vi "make_stim_protocol.vi"(8 "Error in":errorcluster, 10 "Device parameters":T1={"Triggered?"=FALSE, "Shutter channel"="", "Acquisition channels"="", "Acquisition sample rate"=1000.0, "Read chunk size"=100, "Stimulation channel"="Dev1/ao0", "Stimulation sample rate"=100.0} {"Read chunk size" min=100 max=100000; "Acquisition sample rate" min=10.0 max=10000.0 step=10.0; "Stimulation sample rate" min=10.0 max=10000.0}, 11 "Protocol parameters":T2={"Repetitions"=1.0, "ON time"=40.0, "OFF time"=120.0, "Stim onset"=5.0, "Stim frequency"=1.0, "Pulse width"=1.0, "Acquire before ON"=1.0, "Acquire after ON"=1.0, "Sync shutter to acquisition"=TRUE} {"Pulse width" min=0.0001 max=0.1 step=0.01; "Acquire after ON" min=0.0 max=10.0 step=1.0; "Acquire before ON" min=0.0 max=10.0 step=1.0; "Repetitions" min=1.0 max=10.0 step=1.0; "OFF time" min=0.0 max=1000.0; "ON time" min=0.0 max=1000.0; "Stim onset" min=0.0 max=6000.0; "Stim frequency" min=-2.0 max=40.0 step=1.0}) -> (0 "Error out":errorcluster, 2 "Stim array":dbl[](array[numeric]))   [LabVIEW 2010]
uses:
  typedefs/protocol_parameters.ctl
  typedefs/device_parameters.ctl
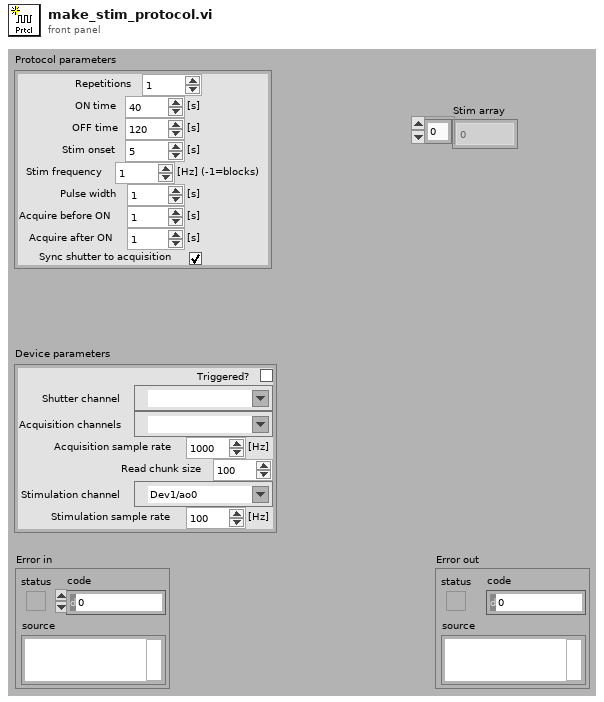
[diagram p1: front panel]
types:
  T1 = typedef "device_parameters.ctl" = cluster{"Triggered?":bool, "Shutter channel":tag, "Acquisition channels":tag, "Acquisition sample rate":dbl, "Read chunk size":i32, "Stimulation channel":tag, "Stimulation sample rate":dbl}
  T2 = typedef "protocol_parameters.ctl" = cluster{"Repetitions":dbl, "ON time":dbl, "OFF time":dbl, "Stim onset":dbl, "Stim frequency":dbl, "Pulse width":dbl, "Acquire before ON":dbl, "Acquire after ON":dbl, "Sync shutter to acquisition":bool}
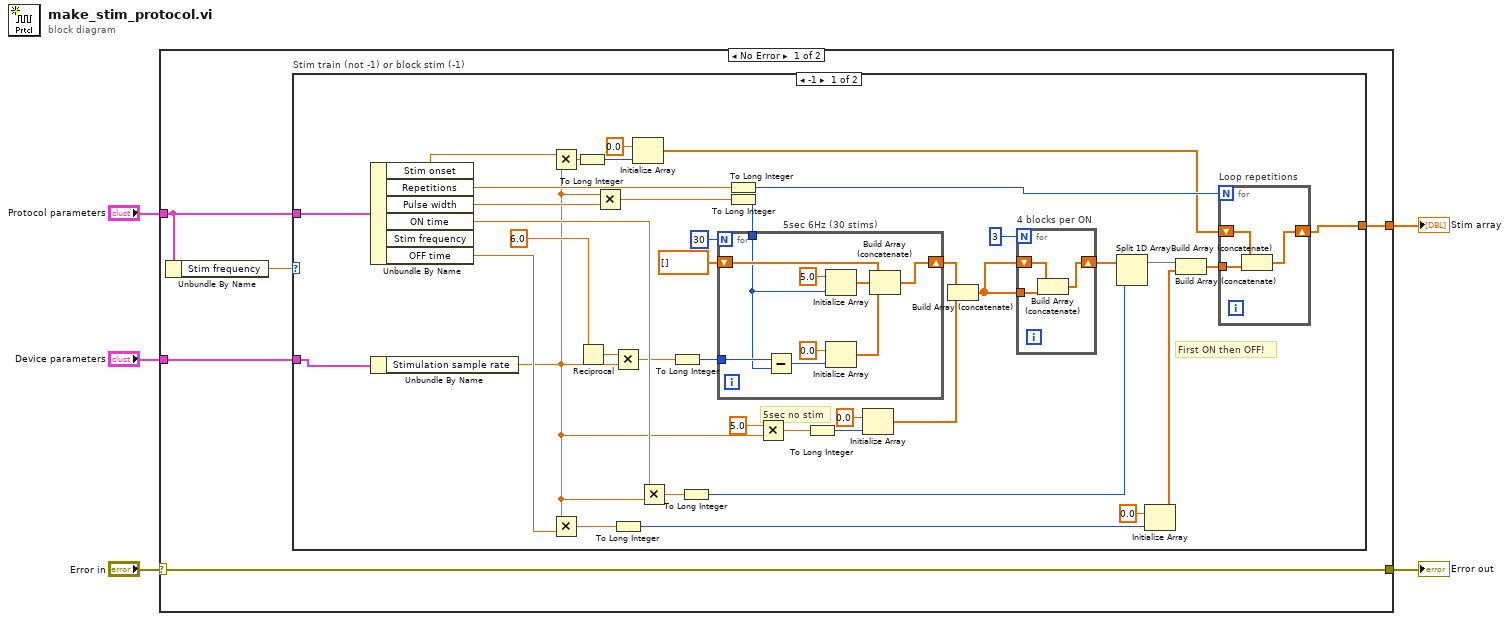
[diagram p0: block diagram]
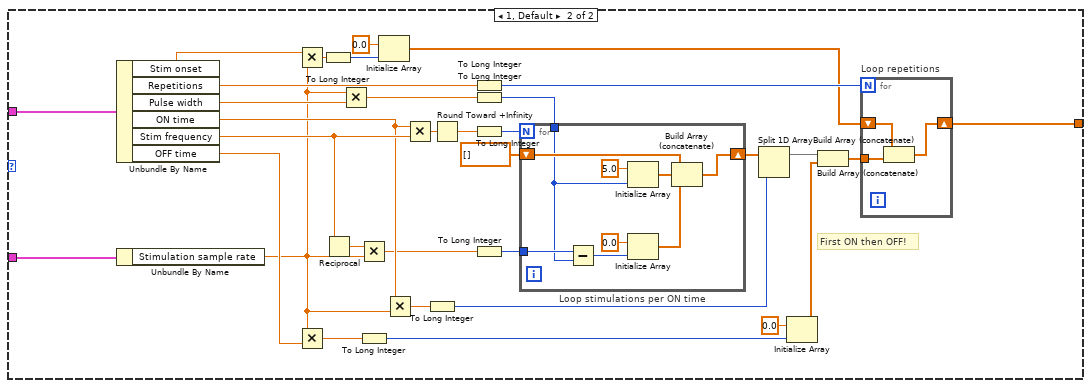
[diagram p2: hidden frame]
diagram:
  n1 = case shown="No Error" "Error in" {
    selector: "Error in" -> [w10 w110]
    tunnel: [w10 w110] -> w4
    tunnel: "Protocol parameters" -> [w7 _]
    tunnel: "Device parameters" -> [w9 _]
    tunnel: [w8 _] -> w1
    frame No Error {
      n2 = Unbundle By Name(w7) -> ("Stim frequency"=w6:dbl)
      n3 = case "Stim train (not -1) or block stim (-1)" shown="-1" w6 {
        tunnel: w7 -> [w25 w97]
        tunnel: w9 -> [w24 w90]
        tunnel: [w11 w77] -> w8
        frame -1 {
          # "5sec no stim"
          # "First ON then OFF!"
          n4 = Unbundle By Name(w25) -> ("Stim onset"=w36:dbl, "Repetitions"=w35:dbl, "Pulse width"=w34:dbl, "ON time"=w47:dbl, "OFF time"=w48:dbl)  [unwired: 1 out]
          n5 = Unbundle By Name(w24) -> ("Stimulation sample rate"=w19:dbl)
          n6 = Multiply(x=w36, y=w19) -> (x*y=w33:dbl)
          n7 = Multiply(x=w19, y=w48) -> (x*y=w41:dbl)
          n8 = To Long Integer(number=w33) -> (32bit integer=w32:i32)
          n9 = Reciprocal(x=6.0 ("y")) -> (1/x=w46:dbl)
          n10 = Multiply(x=w19, y=w34) -> (x*y=w29:dbl)
          n11 = Multiply(x=w46, y=w19) -> (x*y=w31:dbl)
          n12 = To Long Integer(number=w41) -> (32bit integer=w40:i32)
          n13 = Initialize Array(0.0 ("element"), w32) -> (w37:dbl[])
          n14 = Multiply(x=w47, y=w19) -> (x*y=w45:dbl)
          n15 = To Long Integer(number=w31) -> (32bit integer=w30:i32)
          n16 = To Long Integer(number=w45) -> (32bit integer=w43:i32)
          n17 = To Long Integer(number=w35) -> (32bit integer=w39:i32)
          n18 = To Long Integer(number=w29) -> (32bit integer=w28:i32)
          n19 = for "5sec 6Hz (30 stims)" {
            N: 30 -> [_]
            tunnel: w30 -> [w63]
            tunnel: w28 -> [w57]
            shift-right: [w58] -> w14
            shift-left: dbl[] [] -> [w59]
            n20 = Subtract(x=w63, y=w57) -> (x-y=w56:i32)
            n21 = Initialize Array(5.0 ("element"), w57) -> (w61:dbl[])
            n22 = Initialize Array(0.0 ("element"), w56) -> (w60:dbl[])
            n23 = Build Array (concatenate)(w59, w61, w60) -> (w58:dbl[])
          }
          n24 = Multiply(x=5.0, y=w19) -> (x*y=w17:dbl)
          n25 = To Long Integer(number=w17) -> (32bit integer=w18:i32)
          n26 = Initialize Array(0.0 ("element"), w18) -> (w15:dbl[])
          n27 = Build Array (concatenate)(w14, w15) -> (w13:dbl[])
          n28 = for "4 blocks per ON" {
            N: 3 -> [_]
            shift-right: [w50] -> w12
            shift-left: w13 -> [w52]
            tunnel: w13 -> [w51]
            n29 = Build Array (concatenate)(w52, w51) -> (w50:dbl[])
          }
          n30 = Split 1D Array(array=w12, index=w43) -> (first subarray=w26:dbl[])  [unwired: 1 out]
          n31 = Initialize Array(0.0 ("element"), w40) -> (w27:dbl[])
          n32 = Build Array (concatenate)(w26, w27) -> (w38:dbl[])
          n33 = for "Loop repetitions" {
            N: w39 -> [_]
            shift-right: [w53] -> w11
            shift-left: w37 -> [w55]
            tunnel: w38 -> [w54]
            n34 = Build Array (concatenate)(w55, w54) -> (w53:dbl[])
          }
        }
        frame 1, Default {
          # "First ON then OFF!"
          n35 = Unbundle By Name(w97) -> ("Stim onset"=w76:dbl, "Repetitions"=w75:dbl, "Pulse width"=w74:dbl, "ON time"=w91:dbl, "Stim frequency"=w93:dbl, "OFF time"=w92:dbl)
          n36 = Unbundle By Name(w90) -> ("Stimulation sample rate"=w73:dbl)
          n37 = Multiply(x=w76, y=w73) -> (x*y=w72:dbl)
          n38 = Multiply(x=w73, y=w92) -> (x*y=w82:dbl)
          n39 = To Long Integer(number=w72) -> (32bit integer=w71:i32)
          n40 = Reciprocal(x=w93) -> (1/x=w89:dbl)
          n41 = Multiply(x=w73, y=w74) -> (x*y=w68:dbl)
          n42 = Multiply(x=w89, y=w73) -> (x*y=w70:dbl)
          n43 = To Long Integer(number=w82) -> (32bit integer=w81:i32)
          n44 = Initialize Array(0.0 ("element"), w71) -> (w78:dbl[])
          n45 = Multiply(x=w91, y=w73) -> (x*y=w88:dbl)
          n46 = Multiply(x=w91, y=w93) -> (x*y=w95:dbl)
          n47 = To Long Integer(number=w88) -> (32bit integer=w84:i32)
          n48 = Round Toward +Infinity(x=w95) -> (ceil(x): smallest int >= x=w94:dbl)
          n49 = To Long Integer(number=w75) -> (32bit integer=w80:i32)
          n50 = To Long Integer(number=w68) -> (32bit integer=w67:i32)
          n51 = To Long Integer(number=w94) -> (32bit integer=w86:i32)
          n52 = To Long Integer(number=w70) -> (32bit integer=w69:i32)
          n53 = for "Loop stimulations per ON time" {
            N: w86 -> [_]
            tunnel: w69 -> [w108]
            tunnel: w67 -> [w102]
            shift-right: [w103] -> w85
            shift-left: dbl[] [] -> [w104]
            n54 = Subtract(x=w108, y=w102) -> (x-y=w101:i32)
            n55 = Initialize Array(5.0 ("element"), w102) -> (w106:dbl[])
            n56 = Initialize Array(0.0 ("element"), w101) -> (w105:dbl[])
            n57 = Build Array (concatenate)(w104, w106, w105) -> (w103:dbl[])
          }
          n58 = Split 1D Array(array=w85, index=w84) -> (first subarray=w65:dbl[])  [unwired: 1 out]
          n59 = Initialize Array(0.0 ("element"), w81) -> (w66:dbl[])
          n60 = Build Array (concatenate)(w65, w66) -> (w79:dbl[])
          n61 = for "Loop repetitions" {
            N: w80 -> [_]
            shift-right: [w98] -> w77
            shift-left: w78 -> [w100]
            tunnel: w79 -> [w99]
            n62 = Build Array (concatenate)(w100, w99) -> (w98:dbl[])
          }
        }
      }
    }
    frame Error {
    }
  }
  "Error out" <- w4
  "Stim array" <- w1
